vi "GenNumber.vi"() -> (2 "LongitudDelNumero":i32, 3 "RandoNumber":string)   [LabVIEW 2018]
doc: "Genera numeros aleatorios de 8 numeros de longitud, retorna el numero en string y la longitud del numero"
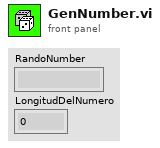
[diagram p1: front panel]
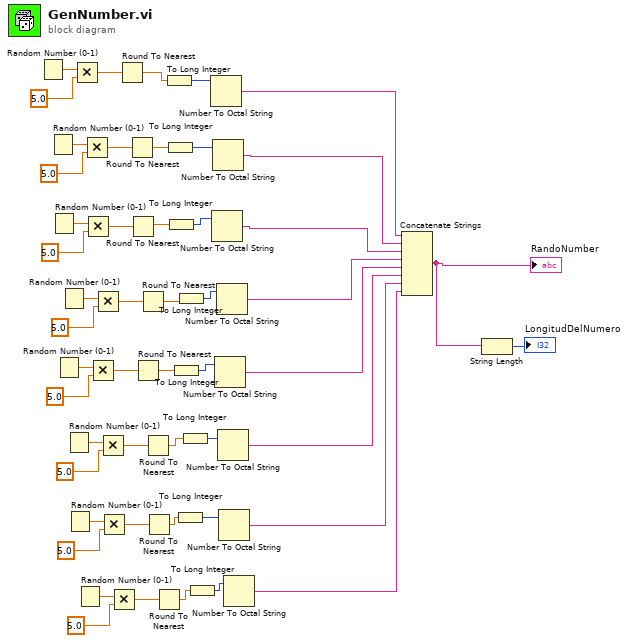
[diagram p0: block diagram]
diagram:
  n1 = Random Number (0-1)() -> (number: 0 to 1=w50:dbl)
  n2 = Random Number (0-1)() -> (number: 0 to 1=w47:dbl)
  n3 = Random Number (0-1)() -> (number: 0 to 1=w44:dbl)
  n4 = Random Number (0-1)() -> (number: 0 to 1=w38:dbl)
  n5 = Random Number (0-1)() -> (number: 0 to 1=w41:dbl)
  n6 = Random Number (0-1)() -> (number: 0 to 1=w35:dbl)
  n7 = Random Number (0-1)() -> (number: 0 to 1=w32:dbl)
  n8 = Multiply(x=w50, y=5.0) -> (x*y=w48:dbl)
  n9 = Random Number (0-1)() -> (number: 0 to 1=w29:dbl)
  n10 = Multiply(x=w47, y=5.0) -> (x*y=w45:dbl)
  n11 = Multiply(x=w44, y=5.0) -> (x*y=w42:dbl)
  n12 = Multiply(x=w38, y=5.0) -> (x*y=w36:dbl)
  n13 = Multiply(x=w41, y=5.0) -> (x*y=w39:dbl)
  n14 = Multiply(x=w35, y=5.0) -> (x*y=w33:dbl)
  n15 = Multiply(x=w32, y=5.0) -> (x*y=w30:dbl)
  n16 = Multiply(x=w29, y=5.0) -> (x*y=w27:dbl)
  n17 = Round To Nearest(number=w48) -> (nearest integer value=w25:dbl)
  n18 = Round To Nearest(number=w45) -> (nearest integer value=w24:dbl)
  n19 = Round To Nearest(number=w42) -> (nearest integer value=w22:dbl)
  n20 = Round To Nearest(number=w36) -> (nearest integer value=w18:dbl)
  n21 = Round To Nearest(number=w39) -> (nearest integer value=w20:dbl)
  n22 = Round To Nearest(number=w33) -> (nearest integer value=w16:dbl)
  n23 = Round To Nearest(number=w30) -> (nearest integer value=w14:dbl)
  n24 = Round To Nearest(number=w27) -> (nearest integer value=w12:dbl)
  n25 = To Long Integer(number=w25) -> (32bit integer=w26:i32)
  n26 = To Long Integer(number=w24) -> (32bit integer=w23:i32)
  n27 = To Long Integer(number=w22) -> (32bit integer=w21:i32)
  n28 = To Long Integer(number=w18) -> (32bit integer=w17:i32)
  n29 = To Long Integer(number=w14) -> (32bit integer=w13:i32)
  n30 = To Long Integer(number=w20) -> (32bit integer=w19:i32)
  n31 = To Long Integer(number=w16) -> (32bit integer=w15:i32)
  n32 = To Long Integer(number=w12) -> (32bit integer=w11:i32)
  n33 = Number To Octal String(2:w26) -> (0:w10:string)  [unwired: 1 in]
  n34 = Number To Octal String(2:w21) -> (0:w8:string)  [unwired: 1 in]
  n35 = Number To Octal String(2:w23) -> (0:w9:string)  [unwired: 1 in]
  n36 = Number To Octal String(2:w17) -> (0:w6:string)  [unwired: 1 in]
  n37 = Number To Octal String(2:w19) -> (0:w7:string)  [unwired: 1 in]
  n38 = Number To Octal String(2:w15) -> (0:w5:string)  [unwired: 1 in]
  n39 = Number To Octal String(2:w13) -> (0:w4:string)  [unwired: 1 in]
  n40 = Number To Octal String(2:w11) -> (0:w3:string)  [unwired: 1 in]
  n41 = Concatenate Strings(w10, w9, w8, w7, w6, w5, w4, w3) -> (w2:string)
  "RandoNumber" <- w2
  n42 = String Length(string=w2) -> (length=→"LongitudDelNumero":i32)
